vi "XY Graph Get-Set Plot Style.vi"(6 "Get (F)/Set":bool, 8 "Error In":errorcluster, 9 "Plot Index":i32 caption="Plot Index (0)", 10 "Plot Style in":T1, 11 "XYGraph in":refnum<vi>) -> (0 "Error Out":errorcluster, 1 "Plot Name":string, 2 "Plot Style out":T1, 3 "Graph Name":string)   [LabVIEW 2021, in "XY Graph Add-Ons.lvlib"]
uses:
  XY Graph Add-Ons.lvlib
  XY Graph Plot Properties.ctl
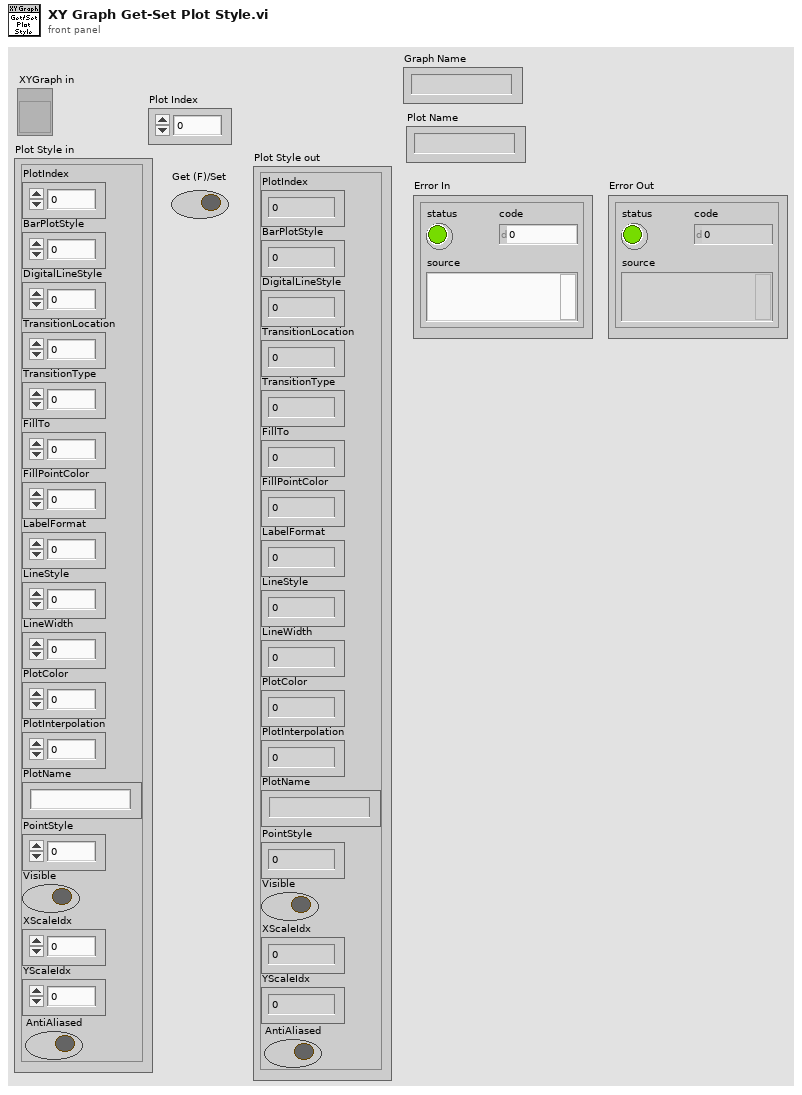
[diagram p1: front panel]
types:
  T1 = typedef "XY Graph Add-Ons.lvlib/XY Graph Plot Properties.ctl" = cluster{"PlotIndex":i32, "BarPlotStyle":u8, "DigitalLineStyle":u8, "TransitionLocation":u8, "TransitionType":u8, "FillTo":i16, "FillPointColor":u32, "LabelFormat":u8, "LineStyle":u8, "LineWidth":u8, "PlotColor":u32, "PlotInterpolation":u8, "PlotName":string, "PointStyle":u8, "Visible":bool, "XScaleIdx":u32, "YScaleIdx":u32, "AntiAliased":bool}
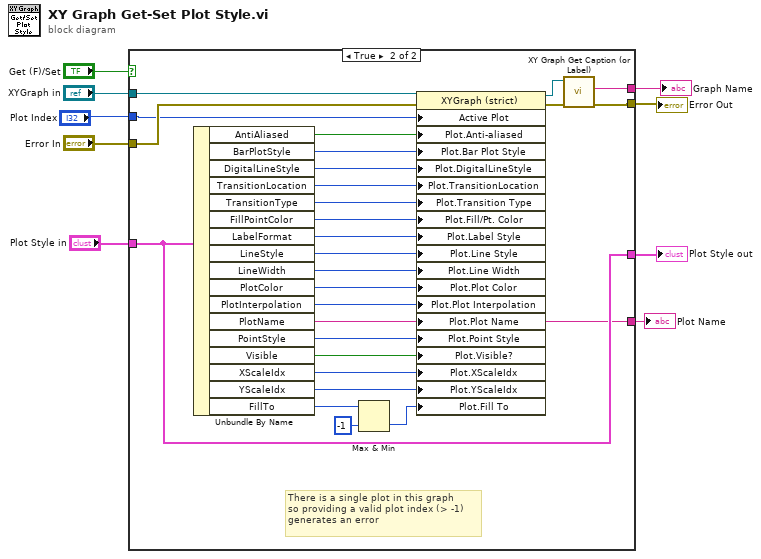
[diagram p0: block diagram]
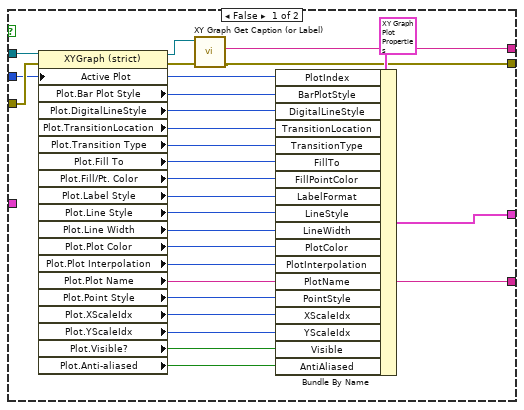
[diagram p2: hidden frame]
diagram:
  n1 = case shown="True" "Get (F)/Set" {
    tunnel: "XYGraph in" -> [w35 w62]
    tunnel: "Plot Index" -> [w32 w60]
    tunnel: "Error In" -> [w34 w61]
    tunnel: [w16 w59] -> w5
    tunnel: [w11 w37] -> w4
    tunnel: "Plot Style in" -> [_ w59]
    tunnel: [w14 w40] -> w2
    tunnel: [w10 w36] -> w1
    frame False {
      n2 = property class="XYGraph (strict)"(reference=w35, error in=w34, "Active Plot"=w32) -> (reference out=w13:refnum<vi>, error out=w12:errorcluster, "Plot.Bar Plot Style"=w31:u8, "Plot.DigitalLineStyle"=w30:u8, "Plot.TransitionLocation"=w29:u8, "Plot.Transition Type"=w27:u8, "Plot.Fill To"=w28:i16, "Plot.Fill/Pt. Color"=w26:u32, "Plot.Label Style"=w25:u8, "Plot.Line Style"=w24:u8, "Plot.Line Width"=w23:u8, "Plot.Plot Color"=w22:u32, "Plot.Plot Interpolation"=w21:u8, "Plot.Plot Name"=w14:string, "Plot.Point Style"=w20:u8, "Plot.XScaleIdx"=w19:u32, "Plot.YScaleIdx"=w18:u32, "Plot.Visible?"=w17:bool, "Plot.Anti-aliased"=w15:bool)
      n3 = call "XY Graph Get Caption (or Label).vi"("error in (no error)"=w12, "XY Graph in"=w13) -> ("error out"=w11:errorcluster, "Caption (or Label) Text"=w10:string)  [unwired: 7 in, 1 out]
      n4 = Bundle By Name(cluster=T1 {"PlotIndex"=0, "BarPlotStyle"=0, "DigitalLineStyle"=0, "TransitionLocation"=0, "TransitionType"=0, "FillTo"=0, "FillPointColor"=0, "LabelFormat"=0, "LineStyle"=0, "LineWidth"=0, "PlotColor"=0, "PlotInterpolation"=0, "PlotName"="", "PointStyle"=0, "Visible"=FALSE, "XScaleIdx"=0, "YScaleIdx"=0, "AntiAliased"=FALSE} ("input cluster"), "PlotIndex"=w32, "BarPlotStyle"=w31, "DigitalLineStyle"=w30, "TransitionLocation"=w29, "TransitionType"=w27, "FillTo"=w28, "FillPointColor"=w26, "LabelFormat"=w25, "LineStyle"=w24, "LineWidth"=w23, "PlotColor"=w22, "PlotInterpolation"=w21, "PlotName"=w14, "PointStyle"=w20, "XScaleIdx"=w19, "YScaleIdx"=w18, "Visible"=w17, "AntiAliased"=w15) -> (w16:T1)
    }
    frame True {
      # "There is a single plot in this graph\nso providing a valid plot index (> -1)\ngenerates an error"
      n5 = Unbundle By Name(w59) -> ("AntiAliased"=w58:bool, "BarPlotStyle"=w57:u8, "DigitalLineStyle"=w56:u8, "TransitionLocation"=w55:u8, "TransitionType"=w54:u8, "FillPointColor"=w53:u32, "LabelFormat"=w49:u8, "LineStyle"=w48:u8, "LineWidth"=w47:u8, "PlotColor"=w46:u32, "PlotInterpolation"=w45:u8, "PlotName"=w40:string, "PointStyle"=w44:u8, "Visible"=w43:bool, "XScaleIdx"=w42:u32, "YScaleIdx"=w41:u32, "FillTo"=w51:i16)
      n6 = Max & Min(x=w51, y=i16 -1 ("Plot.Fill To")) -> (min(x,y)=w50:i16)  [unwired: 1 out]
      n7 = property class="XYGraph (strict)"(reference=w62, error in=w61, "Active Plot"=w60, "Plot.Anti-aliased"=w58, "Plot.Bar Plot Style"=w57, "Plot.DigitalLineStyle"=w56, "Plot.TransitionLocation"=w55, "Plot.Transition Type"=w54, "Plot.Fill/Pt. Color"=w53, "Plot.Label Style"=w49, "Plot.Line Style"=w48, "Plot.Line Width"=w47, "Plot.Plot Color"=w46, "Plot.Plot Interpolation"=w45, "Plot.Plot Name"=w40, "Plot.Point Style"=w44, "Plot.Visible?"=w43, "Plot.XScaleIdx"=w42, "Plot.YScaleIdx"=w41, "Plot.Fill To"=w50) -> (reference out=w39:refnum<vi>, error out=w38:errorcluster)
      n8 = call "XY Graph Get Caption (or Label).vi"("error in (no error)"=w38, "XY Graph in"=w39) -> ("error out"=w37:errorcluster, "Caption (or Label) Text"=w36:string)  [unwired: 7 in, 1 out]
    }
  }
  "Plot Style out" <- w5
  "Error Out" <- w4
  "Plot Name" <- w2
  "Graph Name" <- w1
